vi "ReadSubsetofGFGandWritetoINI.vi"(8 "error in (no error)":errorcluster, 9 "Key Section (_)":string="_", 10 "Variable Names In":string[](array[string]), 11 "Path":path) -> (0 "error out":errorcluster)   [LabVIEW 2017]
doc: "SciScan 1.2 160622\nThis VI reads an INI file and stores all keys in a Generalized Functional Global Variable (GFG). It then monitors updates to the GFG and writes keys back into INI file before closing. Note that the INI file only supports data type DBL or STRING. The GFG can handle any arbitrary data type, but values that are not DBL or STRING are discarded when closing and not written to INI file."
uses:
  <vilib>/Utility/config.llb/Write Key (Double).vi
  <vilib>/Utility/config.llb/Write Key (String).vi
  <vilib>/Utility/config.llb/Write Key (Boolean).vi
  <vilib>/Utility/config.llb/NI_LVConfig.lvlib
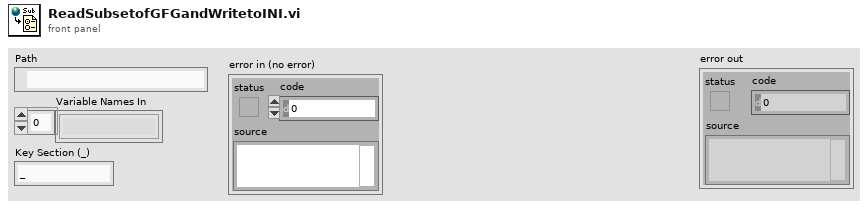
[diagram p1: front panel]
types:
  T1 = typedef "NI_LVConfig.lvlib/Config Data RefNum.ctl" = refnum<k1>
  T2 = typedef "VariantType.lvlib/Type.ctl" = enum8{"Invalid Type", "Void", "I8", "I16", "I32", "I64", "U8", "U16", "U32", "U64", "Single Float", "Double Float", "Extended Float", "Single Complex", "Double Complex", "Extended Complex", "Enum U8", "Enum U16", "Enum U32", "Enum U64", "Single Float With Unit", "Double Float With Unit", "Extended Float With Unit", "Single Complex with Unit", "Double Complex with Unit", "Extended Complex with Unit", "Boolean", "String", "Path", "Picture", "Tag", "Array", "Cluster", "Variant", "LV Variant", "Waveform", "Timestamp", "Digital Waveform", "Digital Data", "ExpressData", "Refnum", "External Data", "VI", "Poly VI", "LabVIEW Class Instance", "Fixed Point"}
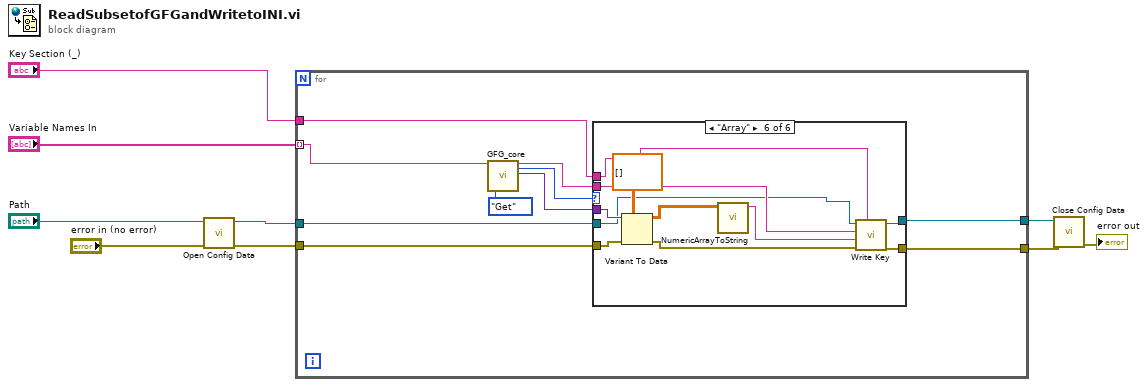
[diagram p0: block diagram]
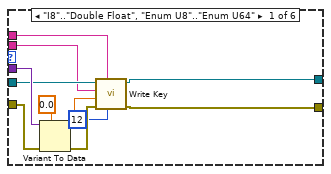
[diagram p2: hidden frame]
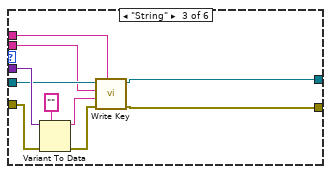
[diagram p4: hidden frame]
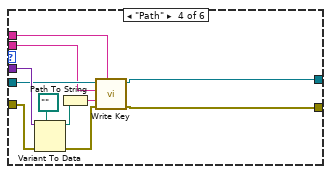
[diagram p5: hidden frame]
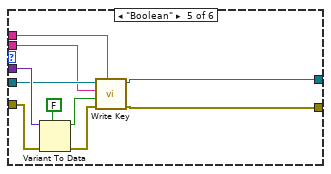
[diagram p6: hidden frame]
diagram:
  n1 = call <vilib>:"Open Config Data.vi"("error in (no error)"="error in (no error)", "configuration file path"="Path") -> ("error out"=w7:errorcluster, "refnum"=w8:T1)  [unwired: 7 in, 1 out]
  n2 = for {
    tunnel: [w18] -> w4
    tunnel: w8 -> [w17]
    tunnel: w7 -> [w19]
    tunnel: [w16] -> w5
    tunnel: "Variable Names In" -> [w14] mode=indexing
    tunnel: "Key Section (_)" -> [w15]
    n3 = call "GFG_core.vi"("Variable Name in"=w14, "Action"=enum16{"Init", "Set", "Get"}."Get") -> ("Variable Name Out"=w10:string, "Data Type Out"=w12:T2, "Variant Out"=w11:variant)  [unwired: 11 in, 4 out]
    n4 = case shown="\"Array\"" w12 {
      tunnel: w11 -> [w29 _ w42 w53 w63 w74]
      tunnel: [w26 w32 w39 w51 w60 w70] -> w18
      tunnel: w19 -> [w25 w32 w38 w50 w59 w72]
      tunnel: w17 -> [w24 w31 w37 w49 w58 w66]
      tunnel: [w23 w31 w36 w48 w57 w65] -> w16
      tunnel: w10 -> [w22 _ w35 w47 w56 w67]
      tunnel: w15 -> [w21 _ w34 w46 w55 w64]
      frame "I8".."Double Float", "Enum U8".."Enum U64" {
        n5 = Variant To Data(error in=w25, type=0.0, Variant=w29) -> (data=w28:dbl, error out=w27:errorcluster)
        n6 = call-poly <vilib>:"Write Key.vi"("precision (6)"=i16 12, "section"=w21, "error in (no error)"=w27, "value"=w28, "key"=w22, "refnum"=w24) -> ("error out"=w26:errorcluster, "refnum out"=w23:T1)  [unwired: 3 in, 1 out]
      }
      frame Default {
      }
      frame "String" {
        n7 = Variant To Data(error in=w38, type="" ("Variable Name Out"), Variant=w42) -> (data=w41:string, error out=w40:errorcluster)
        n8 = call-poly <vilib>:"Write Key.vi"("section"=w34, "error in (no error)"=w40, "value"=w41, "key"=w35, "refnum"=w37) -> ("error out"=w39:errorcluster, "refnum out"=w36:T1)  [unwired: 4 in, 1 out]
      }
      frame "Path" {
        n9 = Variant To Data(error in=w50, type=path "" ("configuration file path 2"), Variant=w53) -> (data=w43:path, error out=w52:errorcluster)
        n10 = Path To String(path=w43) -> (string=w44:string)
        n11 = call-poly <vilib>:"Write Key.vi"("section"=w46, "error in (no error)"=w52, "value"=w44, "key"=w47, "refnum"=w49) -> ("error out"=w51:errorcluster, "refnum out"=w48:T1)  [unwired: 4 in, 1 out]
      }
      frame "Boolean" {
        n12 = Variant To Data(error in=w59, type=FALSE, Variant=w63) -> (data=w62:bool, error out=w61:errorcluster)
        n13 = call-poly <vilib>:"Write Key.vi"("section"=w55, "error in (no error)"=w61, "value"=w62, "key"=w56, "refnum"=w58) -> ("error out"=w60:errorcluster, "refnum out"=w57:T1)  [unwired: 4 in, 1 out]
      }
      frame "Array" {
        n14 = Variant To Data(error in=w72, type=dbl[][] [], Variant=w74) -> (data=w69:dbl[][], error out=w71:errorcluster)
        n15 = call "NumericArrayToString.vi"("Array In"=w69) -> ("String Out"=w68:string)  [unwired: 10 in]
        n16 = call-poly <vilib>:"Write Key.vi"("section"=w64, "error in (no error)"=w71, "value"=w68, "key"=w67, "refnum"=w66) -> ("error out"=w70:errorcluster, "refnum out"=w65:T1)  [unwired: 4 in, 1 out]
      }
    }
  }
  n17 = call <vilib>:"Close Config Data.vi"("error in (no error)"=w4, "refnum"=w5) -> ("error out"=→"error out":errorcluster)  [unwired: 8 in, 1 out]
